vi "Differential Spikes chopper.vi"(4 "Spikes Array In":cluster{"Index":i32, "max value":sgl}[](array[cluster]), 5 "Analysis Info cluster In":T1={"Colour"=0, "Inst type"=enum."Pitot-static tube", "Inst name"="Manometer voltage", "Symbol"="U", "Code name"="", "Extra Info"="U", "Inst Array"=enum."PWA", "U"=0.0, "u^2"=0.0, "u^3"=0.0, "u^4"=0.0, "Skew_u"=0.0, "Kurt_u"=0.0, "Sd Error in Mean"=0.0, "% u'/U"=0.0, "X"=0.0, "Y"=0.0, "Z"=0.0, "Timescale integral Estimate"=0.0, "Sd Error in Variance"=0.0, "Calib File"=path "", "Calib Constants"=[], "Output Position"=FALSE, "Stats"=enum."None", "Av Sampling Rate"=0.0, "Av No of Samples"=0.0, "Total Meas Time (s)"=0.0, "OrigChName"="", "Max value"=0.0, "Min value"=0.0, "Req Sample Rate Hz"=0.0, "Sync Delay Time (s)"=0.0, "Ch No"=0, "Device"="", "Use Latest Calib"=FALSE, "Port"="", "Metadata Ch Names"=[], "Metadata Ch Values"=[], "Label"="", "chState"=enum."Solo", "Point Drift"=0.0, "inputConfig"=""} {"Kurt_u" format="%_3g"; "u^4" format="%_3g"; "u^3" format="%_3g"; "Sd Error in Variance" format="%_3g"; "u^2" format="%_3g"; "Sd Error in Mean" format="%_3g"; "U" format="%_3g"; "Sync Delay Time (s)" format="%.4f"; "Total Meas Time (s)" format="%_5g"; "Skew_u" format="%_3g"; "% u'/U" format="%_3g"}, 6 "Average Sampling Rate":sgl, 7 "C Trace":dbl[](array[numeric])) -> (0 "Spikes Array Out":cluster{"Index":i32, "max value":dbl}[](array[cluster]), 1 "No of Removed spikes":i32, 3 "Filtered Time Trace":sgl[](array[numeric]))   [LabVIEW 2022 SP3]
uses:
  Controls/Analysis_info_cluster.ctl
  Controls/Inst_type.ctl
  Controls/Instrument_Array.ctl
  Controls/channelState.ctl
panel:
  in  "Factor 2":sgl=2.5
  out "Min Spike Length":i32
  out "Spike Length":i32
  in  "Factor":sgl=1.5
  in  "p":sgl=0.97
  out "percentile":sgl
  out "Spike 2nd  All":sgl[](graph)
  out "Inst name":string
  in  "Play thro":bool
  out "Start time (Sec)":sgl
  in  "Display removed spikes":bool
  out "Potential spikes2":cluster{"Start Index":i32, "End Index":i32}[](array[cluster])
  out "Spikes1":cluster{"Start Index":i32, "End Index":i32}[](array[cluster])
  out "element":cluster{"Start Index":i32, "End Index":i32}
  in  "stop":bool
  in  "Desired index":i32 min=0
  out "Spike C":sgl[][](graph)
  out "Spike 2nd Derivative":sgl[](graph)
  out "Spikes 3":cluster{"Start Index":i32, "End Index":i32}[](array[cluster])
  out "C Threshold":sgl
  in  "Point info":cluster{"Start Index":i32, "End Index":i32}
  out "Derivative Theshold 1":sgl
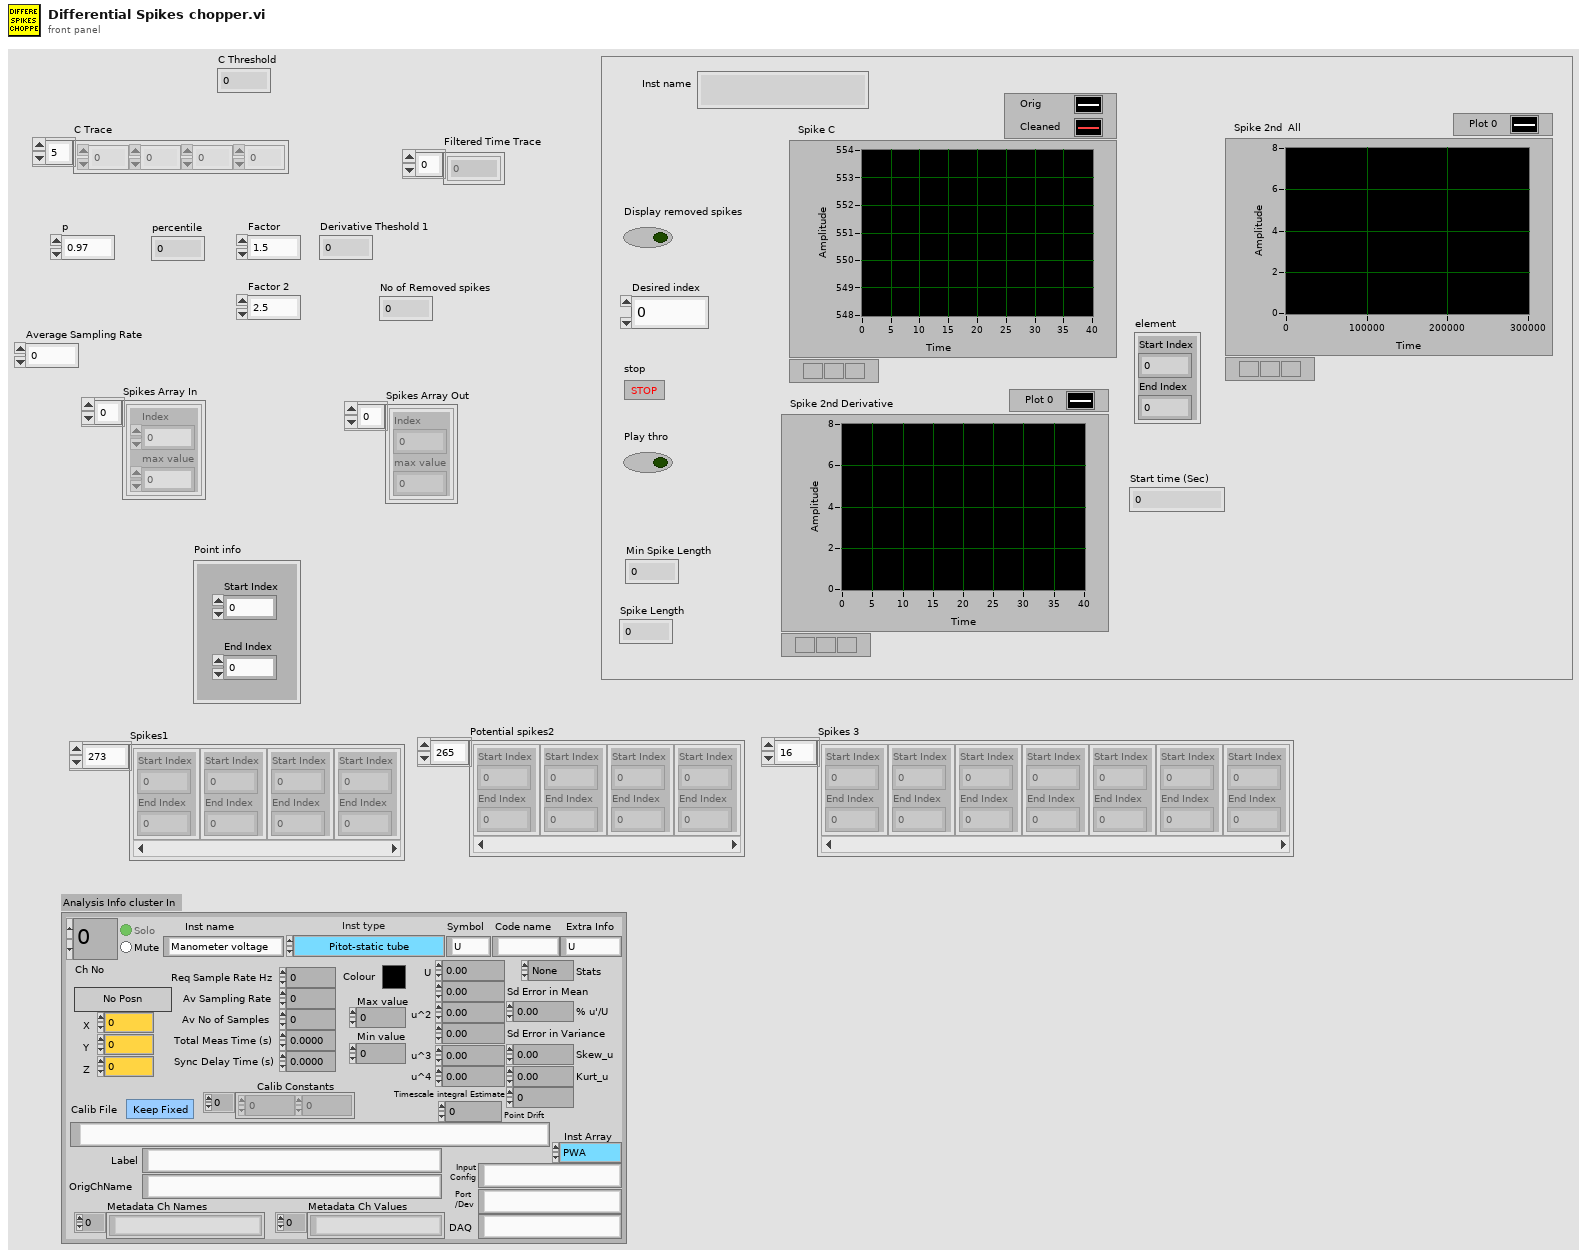
[diagram p1: front panel]
types:
  T1 = typedef "Analysis_info_cluster.ctl" = cluster{"Colour":u32, "Inst type":T2, "Inst name":string, "Symbol":string, "Code name":string, "Extra Info":string, "Inst Array":T3, "U":dbl, "u^2":dbl, "u^3":dbl, "u^4":dbl, "Skew_u":dbl, "Kurt_u":dbl, "Sd Error in Mean":dbl, "% u'/U":dbl, "X":dbl, "Y":dbl, "Z":dbl, "Timescale integral Estimate":dbl, "Sd Error in Variance":dbl, "Calib File":path, "Calib Constants":dbl[], "Output Position":bool, "Stats":enum16{"None", "Basic", "Full"}, "Av Sampling Rate":dbl, "Av No of Samples":dbl, "Total Meas Time (s)":dbl, "OrigChName":string, "Max value":dbl, "Min value":dbl, "Req Sample Rate Hz":dbl, "Sync Delay Time (s)":dbl, "Ch No":i16, "Device":string, "Use Latest Calib":bool, "Port":string, "Metadata Ch Names":string[], "Metadata Ch Values":string[], "Label":string, "chState":T4, "Point Drift":dbl, "inputConfig":string}
  T2 = typedef "Inst_type.ctl" = enum16{"Raw voltage", "Raw with zero offsetting", "Propeller anemometer", "Pressure Transducer", "Pitot-static tube", "Hot wire", "Cross wire 1", "Cross wire 2", "Generic Linear", "Generic Polynomial", "Generic BackPoly", "Fast FID", "Thermocouple", "Cold wire", "Pulsed Wire", "LDA Vel", "LDA Tran time", "LDA Arr time", "Microphone"}
  T3 = typedef "Instrument_Array.ctl" = enum16{"PWA", "LDA", "Analogue"}
  T4 = typedef "channelState.ctl" = enum32{"No Selection", "Solo", "Mute"}
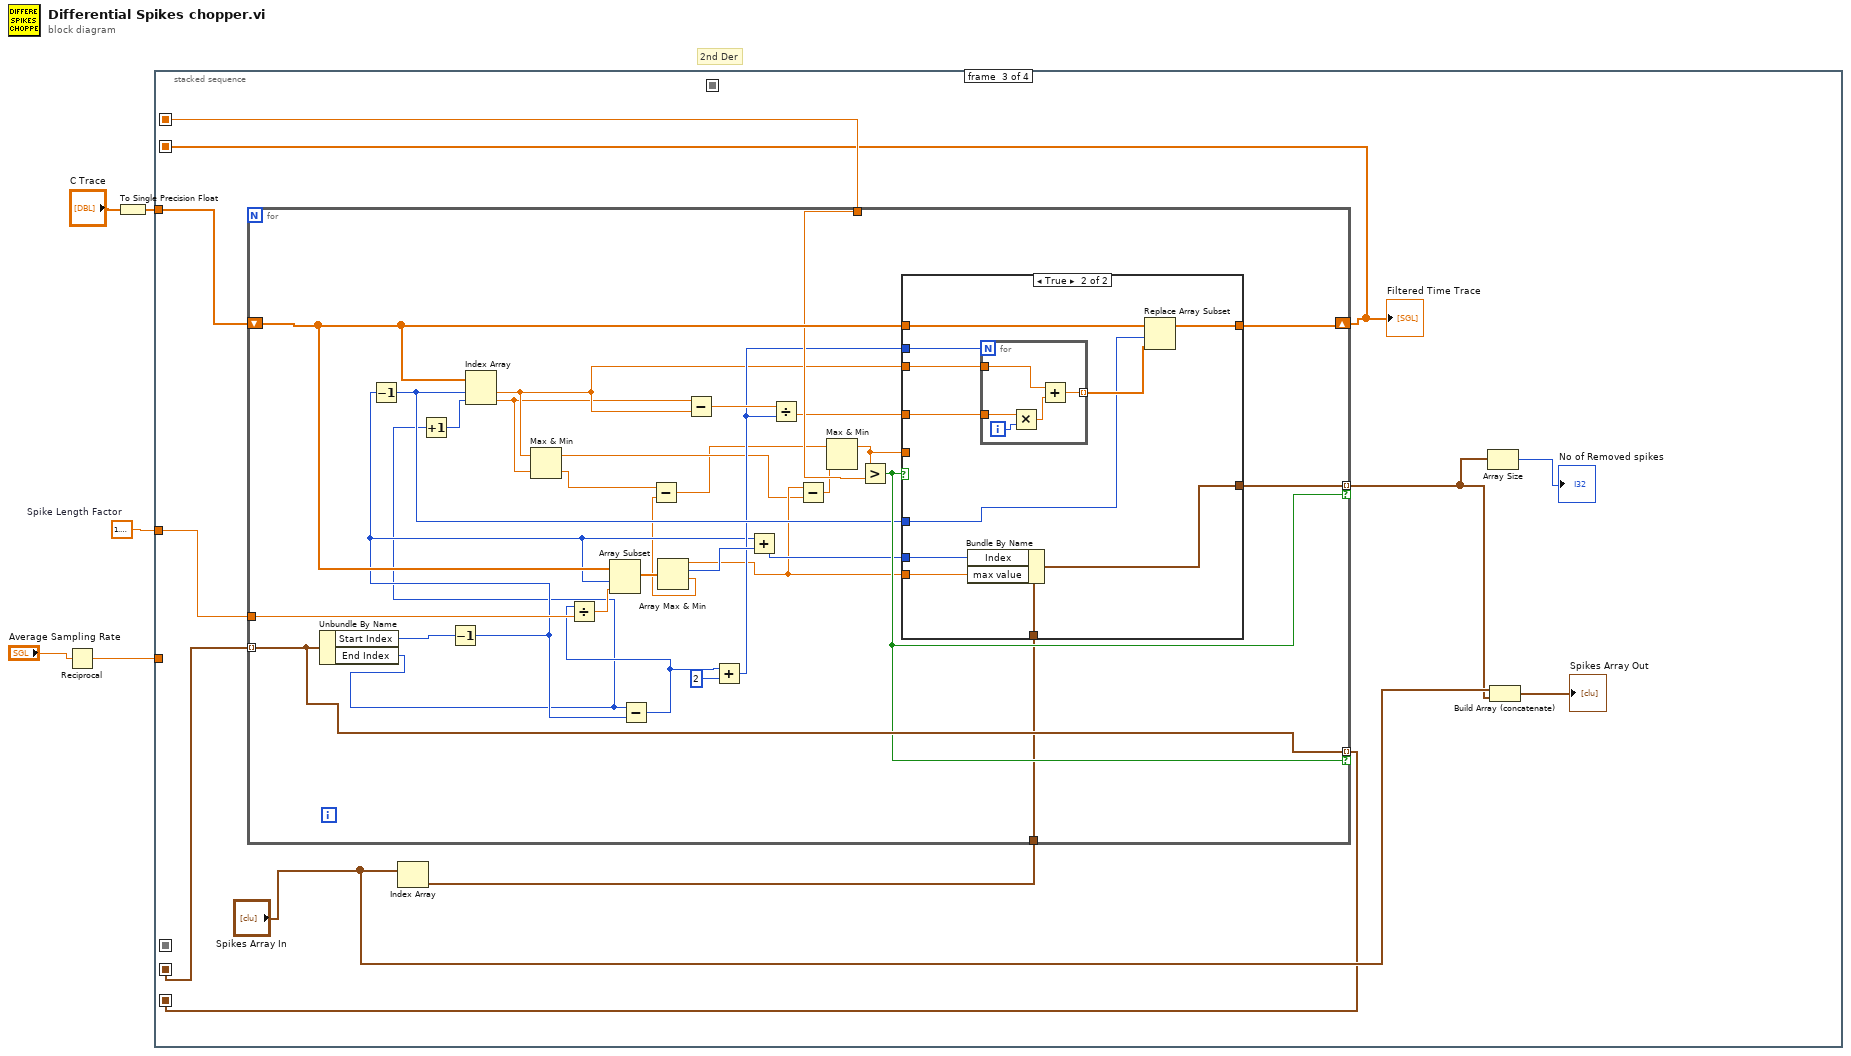
[diagram p0: block diagram]
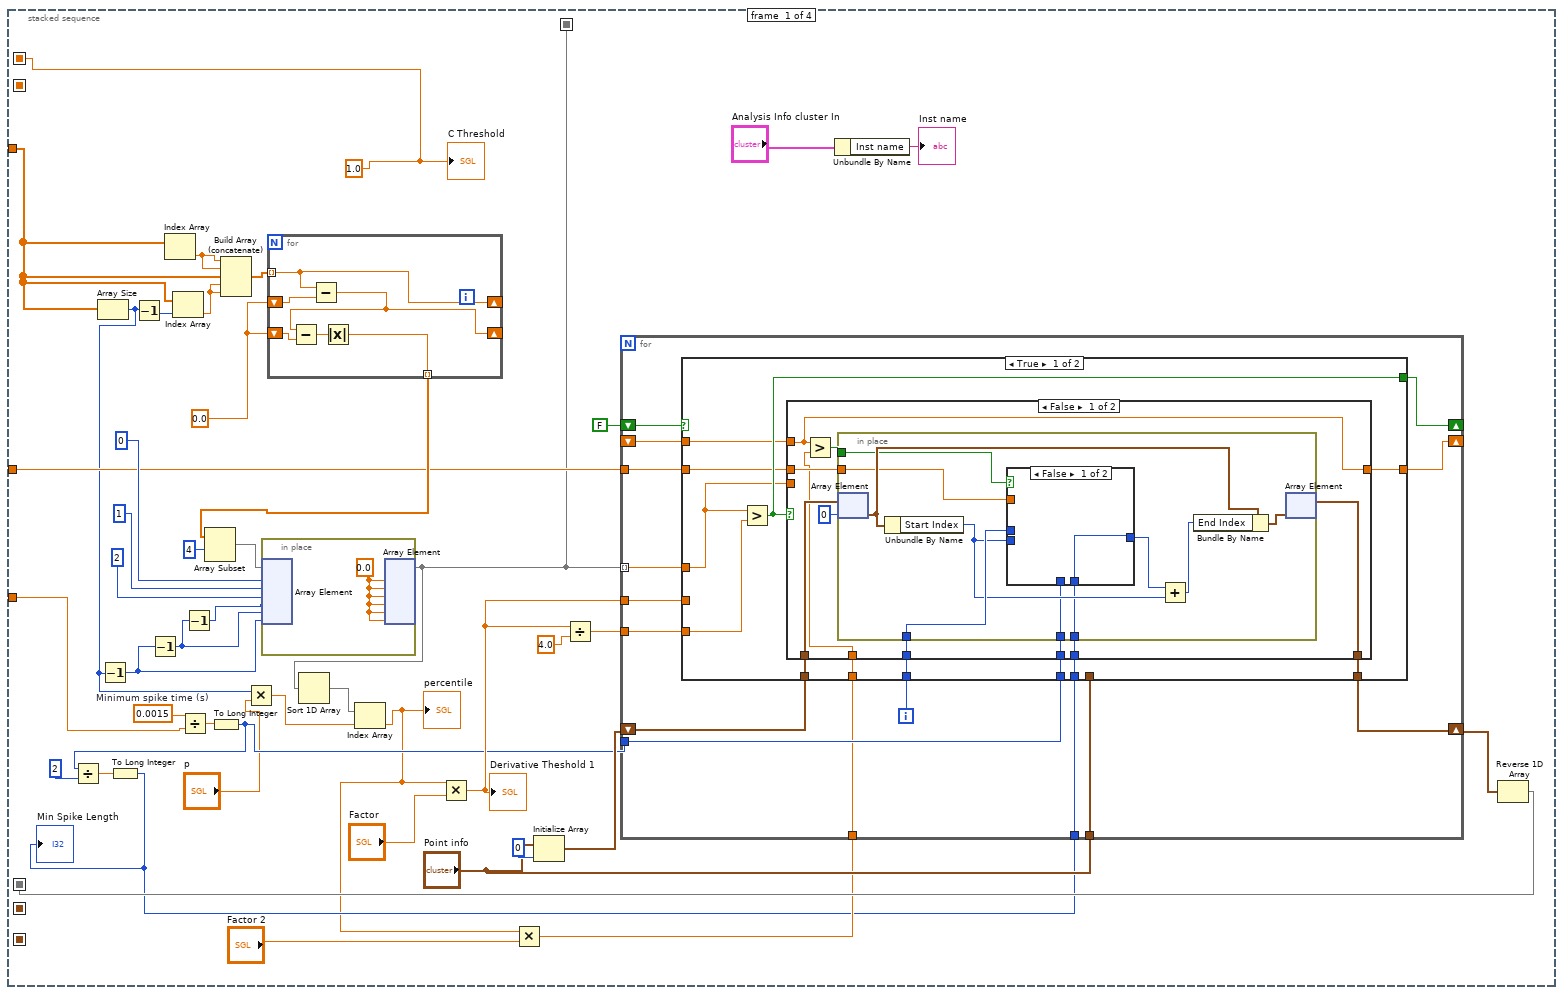
[diagram p2: hidden frame]
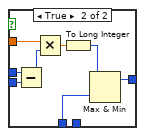
[diagram p3: hidden frame]
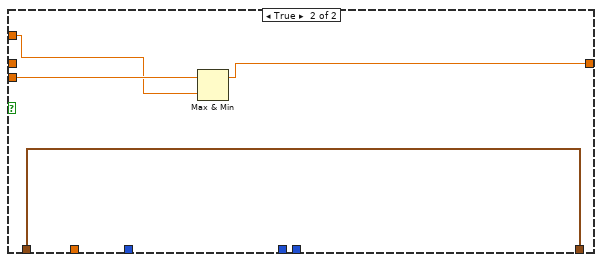
[diagram p4: hidden frame]
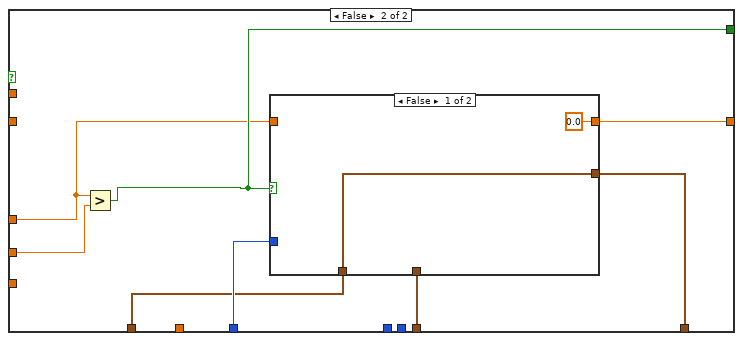
[diagram p5: hidden frame]
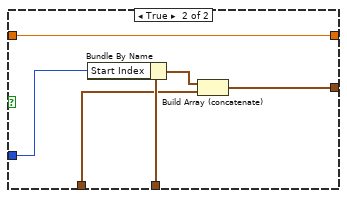
[diagram p6: hidden frame]
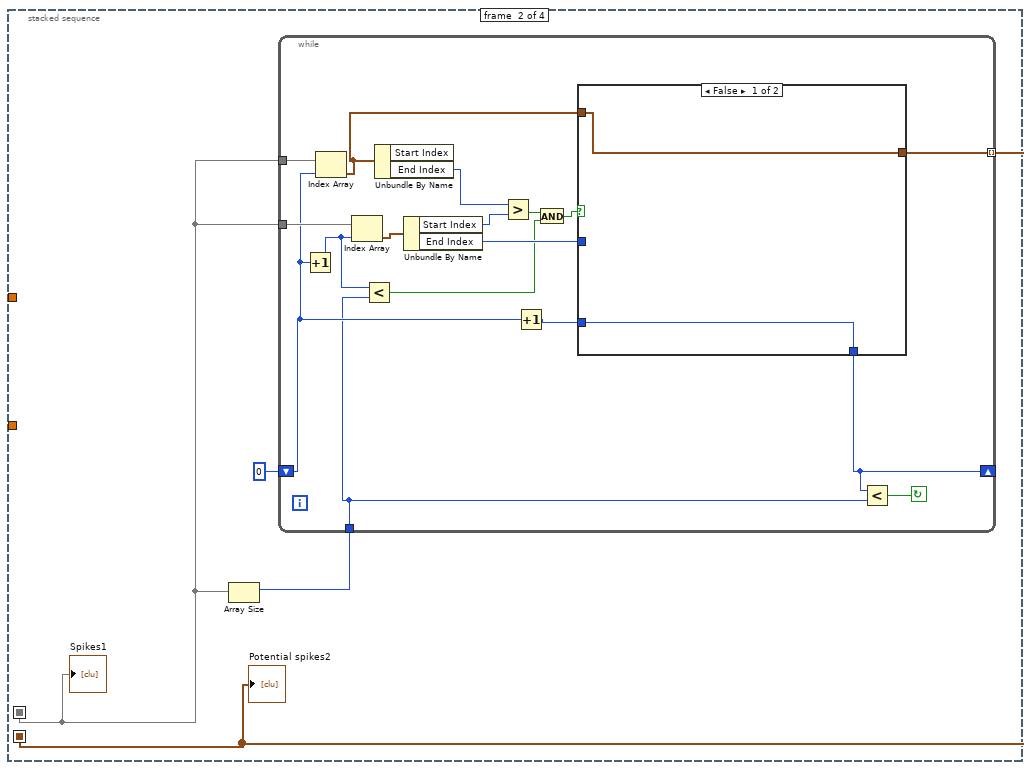
[diagram p7: hidden frame]
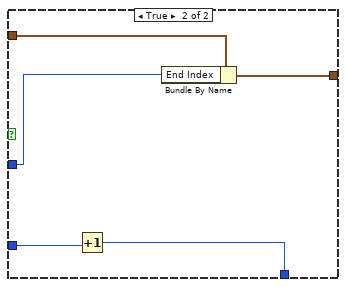
[diagram p8: hidden frame]
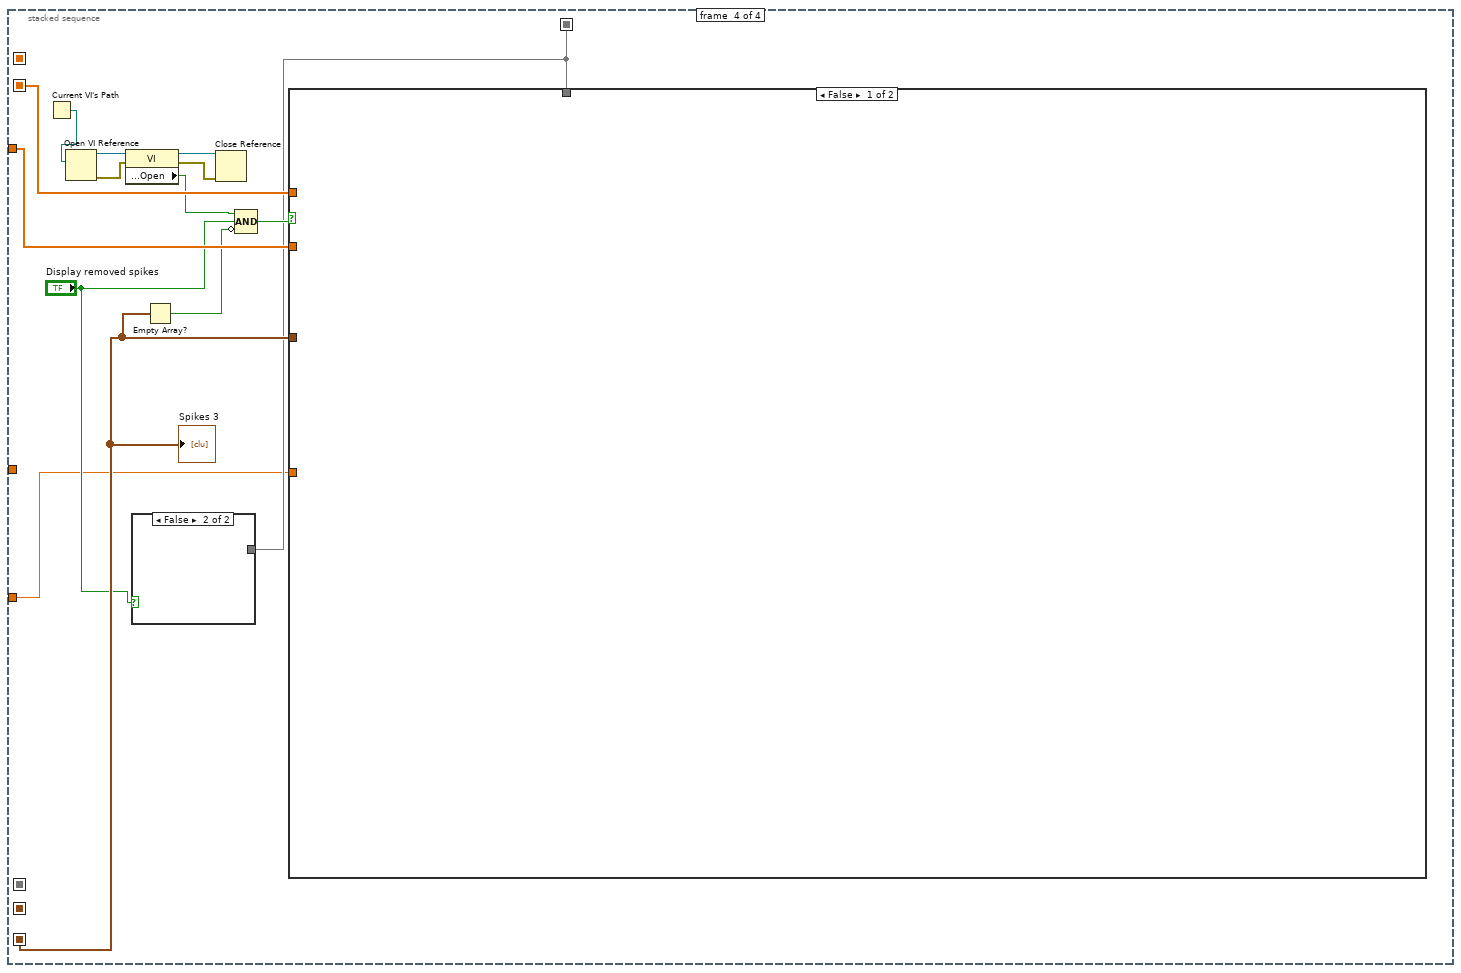
[diagram p10: hidden frame]
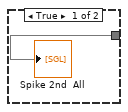
[diagram p11: hidden frame]
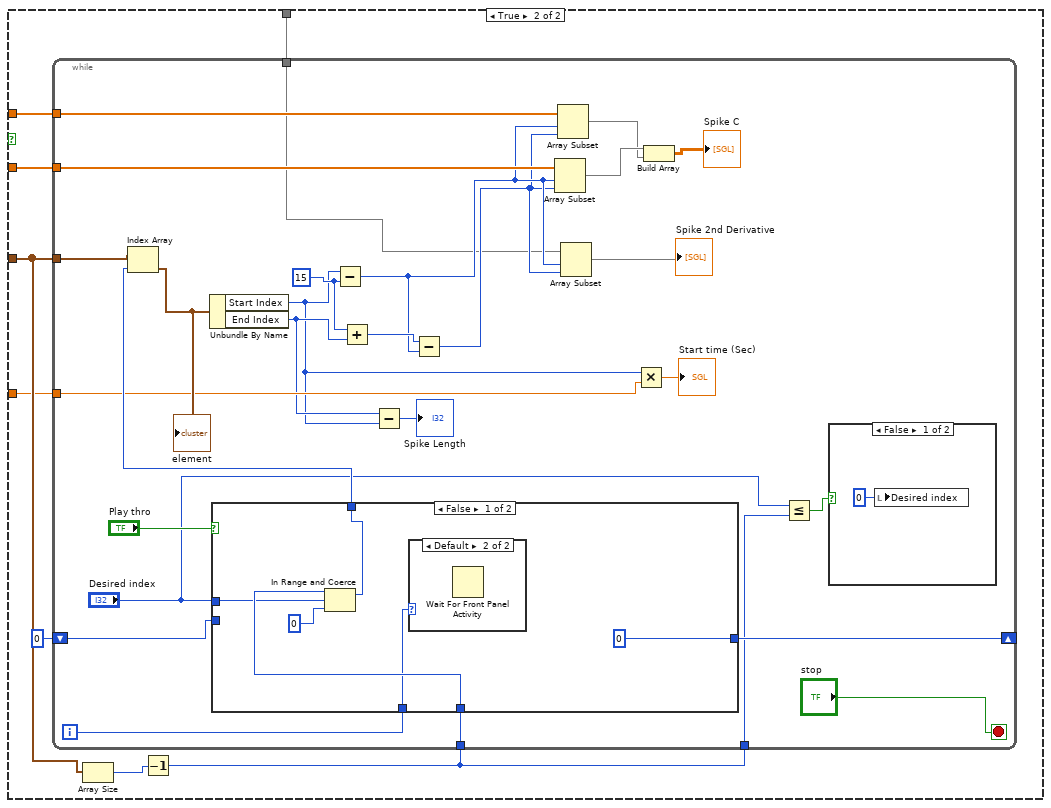
[diagram p12: hidden frame]
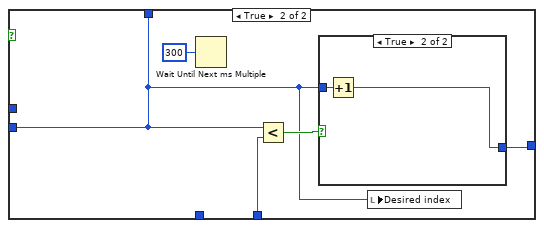
[diagram p15: hidden frame]
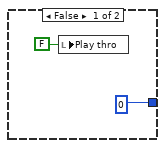
[diagram p16: hidden frame]
diagram:
  w4 = sgl 1.9  # Spike Length Factor
  # "2nd Der"
  n1 = Reciprocal(x="Average Sampling Rate") -> (1/x=w2:sgl)
  n2 = To Single Precision Float(number="C Trace") -> (single precision float=w1:sgl[])
  n3 = stacked-sequence {
    seq-local: [w29 _ _ _] -> [_ w135 _ _]
    seq-local: [w18 _ _ _] -> [_ _ w167 _]
    seq-local: [_ _ w164 _] -> [_ _ _ w226]
    seq-local: [_ _ w163 _] -> [_ _ _ w233]
    seq-local: [w11 _ _ _] -> [_ _ _ w222]
    seq-local: [_ w134 _ _] -> [_ _ w162 _]
    tunnel: w1 -> [w34 _ w171 w234]
    tunnel: w4 -> [w28 _ w161 _]
    tunnel: w2 -> [w20 _ _ w221]
    frame #0 {
      w18 = sgl 1.0 ("C Threshold")
      w21 = 0.0015  # Minimum spike time (s)
      w44 = sgl 0.0
      n4 = Array Size(array=w34) -> (size(s)=w9:i32)
      n5 = Decrement(x=w9) -> (x-1=w37:i32)
      n6 = Decrement(x=w9) -> (x-1=w46:i32)
      n7 = Decrement(x=w37) -> (x-1=w35:i32)
      n8 = Index Array(array=w34) -> (element=w47:sgl)  [unwired: 1 in]
      n9 = Index Array(array=w34, index=w46) -> (element=w45:sgl)
      n10 = Divide(x=w21, y=w20) -> (x/y=w19:dbl)
      n11 = Decrement(x=w35) -> (x-1=w36:i32)
      n12 = To Long Integer(number=w19) -> (32bit integer=w17:i32)
      n13 = Divide(x=w17, y=2) -> (x/y=w15:dbl)
      n14 = To Long Integer(number=w15) -> (32bit integer=w12:i32)
      "Min Spike Length" <- w12
      n15 = Build Array (concatenate)(w47, w47, w34, w45, w45) -> (w48:sgl[])
      n16 = Multiply(x=w9, y="p") -> (x*y=w7:sgl)
      n17 = for {
        shift-right: [w53] -> _
        shift-left: w44 -> [w56]
        tunnel: w48 -> [w53] mode=indexing
        tunnel: [w51] -> w39 mode=indexing
        shift-right: [w52] -> _
        shift-left: w44 -> [w55]
        n18 = Subtract(x=w53, y=w56) -> (x-y=w52:sgl)
        n19 = Subtract(x=w52, y=w55) -> (x-y=w54:sgl)
        n20 = Absolute Value(x=w54) -> (abs(x)=w51:sgl)
      }
      n21 = Array Subset(array=w39, index=4) -> (w38:sgl[])  [unwired: 1 in]
      n22 = in-place {
        w50 = sgl 0.0 ("element")
        n23 = in-place-array #1(w38, 0, 1, 2, w36, w35, w37) -> ()  [unwired: 6 out]
        n24 = in-place-array #1(w50, w50, w50, w50, w50, w50) -> (w11:sgl[])  [unwired: 6 out]
      }
      n25 = Sort 1D Array(array=w11) -> (sorted array=w8:sgl[])
      n26 = Index Array(array=w8, index=w7) -> (element=w6:sgl)
      "percentile" <- w6
      n27 = Multiply(x=w6, y="Factor") -> (x*y=w24:sgl)
      "Derivative Theshold 1" <- w24
      n28 = Multiply(x=w6, y="Factor 2") -> (x*y=w13:sgl)
      n29 = Initialize Array("Point info", 0 ("dimension size")) -> (w32:cluster{"Start Index":i32, "End Index":i32}[])
      n30 = Divide(x=w24, y=sgl 4.0) -> (x/y=w23:sgl)
      n31 = for {
        shift-right: [w67] -> _
        shift-left: FALSE -> [w70]
        tunnel: w11 -> [w71] mode=indexing
        tunnel: w24 -> [w69]
        shift-right: [w64] -> w30
        shift-left: w32 -> [w65]
        tunnel: "Point info" -> [w66]
        tunnel: w28 -> [w63]
        tunnel: w23 -> [w62]
        tunnel: w17 -> [w61]
        shift-right: [w60] -> _
        shift-left: _ -> [w59]
        tunnel: w13 -> [w58]
        tunnel: w12 -> [w57]
        i -> [w68]
        n32 = case shown="True" w70 {
          tunnel: [w80 w119] -> w67
          tunnel: w71 -> [w76 w117]
          tunnel: w69 -> [_ w124]
          tunnel: w68 -> [w81 w123]
          tunnel: w66 -> [_ w122]
          tunnel: w65 -> [w83 w121]
          tunnel: [w82 w120] -> w64
          tunnel: w63 -> [w79 _]
          tunnel: w62 -> [w78 _]
          tunnel: w61 -> [w77 _]
          tunnel: [w74 w118] -> w60
          tunnel: w59 -> [w75 _]
          tunnel: w58 -> [w73 _]
          tunnel: w57 -> [w72 _]
          frame True {
            n33 = Greater?(x=w76, y=w78) -> (0:w80:bool)
            n34 = case shown="False" w80 {
              tunnel: w81 -> [w89 _]
              tunnel: w83 -> [w93 w116]
              tunnel: [w92 w116] -> w82
              tunnel: w79 -> [w90 _]
              tunnel: w77 -> [w88 _]
              tunnel: w76 -> [_ w115]
              tunnel: w75 -> [w84 w114]
              tunnel: [w84 w113] -> w74
              tunnel: w73 -> [w87 _]
              tunnel: w72 -> [w85 _]
              frame False {
                n35 = Greater?(x=w84, y=w87) -> (0:w86:bool)
                n36 = in-place {
                  in-place-border: w90 -> [w101]
                  in-place-border: w89 -> [w100]
                  in-place-border: w88 -> [w97]
                  in-place-border: w86 -> [w95]
                  in-place-border: w85 -> [w94]
                  n37 = in-place-array #2(w93, 0) -> (w103:cluster{"Start Index":i32, "End Index":i32})
                  n38 = Unbundle By Name(w103) -> ("Start Index"=w99:i32)
                  n39 = case shown="False" w95 {
                    tunnel: w101 -> [_ w110]
                    tunnel: w100 -> [_ w109]
                    tunnel: w99 -> [_ w108]
                    tunnel: w97 -> [_ w106]
                    tunnel: [w104 w105] -> w96
                    tunnel: w94 -> [w104 _]
                    frame False {
                    }
                    frame True {
                      n40 = Subtract(x=w109, y=w108) -> (x-y=w111:i32)
                      n41 = Multiply(x=w110, y=w111) -> (x*y=w112:sgl)
                      n42 = To Long Integer(number=w112) -> (32bit integer=w107:i32)
                      n43 = Max & Min(x=w107, y=w106) -> (max(x,y)=w105:i32)  [unwired: 1 out]
                    }
                  }
                  n44 = Add(x=w96, y=w99) -> (x+y=w98:i32)
                  n45 = Bundle By Name(cluster=w103, "End Index"=w98) -> (w102:cluster{"Start Index":i32, "End Index":i32})
                  n46 = in-place-array #2(w102) -> (w92:cluster{"Start Index":i32, "End Index":i32}[])  [unwired: 1 out]
                }
              }
              frame True {
                n47 = Max & Min(x=w115, y=w114) -> (max(x,y)=w113:sgl)  [unwired: 1 out]
              }
            }
          }
          frame False {
            n48 = Greater?(x=w117, y=w124) -> (0:w119:bool)
            n49 = case shown="False" w119 {
              tunnel: w123 -> [_ w132]
              tunnel: w122 -> [_ w130]
              tunnel: w121 -> [w126 w129]
              tunnel: [w126 w128] -> w120
              tunnel: [sgl 0.0 w127] -> w118
              tunnel: w117 -> [_ w127]
              frame False {
              }
              frame True {
                n50 = Bundle By Name(cluster=w130, "Start Index"=w132) -> (w131:cluster{"Start Index":i32, "End Index":i32})
                n51 = Build Array (concatenate)(w131, w129) -> (w128:cluster{"Start Index":i32, "End Index":i32}[])
              }
            }
          }
        }
      }
      n52 = Unbundle By Name("Analysis Info cluster In") -> ("Inst name"=→"Inst name":string)
      n53 = Reverse 1D Array(array=w30) -> (reversed array=w29:cluster{"Start Index":i32, "End Index":i32}[])
      "C Threshold" <- w18
    }
    frame #1 {
      n54 = Array Size(array=w135) -> (size(s)=w133:i32)
      n55 = while {
        tunnel: w135 -> [w146]
        tunnel: w135 -> [w153]
        tunnel: [w148] -> w134 mode=indexing
        shift-right: [w143] -> _
        shift-left: 0 -> [w145]
        tunnel: w133 -> [w137]
        stop <- w142 continue-if-true
        n56 = Increment(x=w145) -> (x+1=w141:i32)
        n57 = Index Array(array=w146, index=w145) -> (element=w147:cluster{"Start Index":i32, "End Index":i32})
        n58 = Index Array(array=w153, index=w141) -> (element=w152:cluster{"Start Index":i32, "End Index":i32})
        n59 = Less?(x=w141, y=w137) -> (x < y?=w139:bool)
        n60 = Unbundle By Name(w147) -> ("End Index"=w151:i32)  [unwired: 1 out]
        n61 = Unbundle By Name(w152) -> ("Start Index"=w150:i32, "End Index"=w149:i32)
        n62 = Greater?(x=w151, y=w150) -> (0:w140:bool)
        n63 = Increment(x=w145) -> (x+1=w144:i32)
        n64 = And(x=w140, y=w139) -> (x .and. y?=w138:bool)
        n65 = case shown="False" w138 {
          tunnel: w147 -> [w154 w160]
          tunnel: w149 -> [_ w159]
          tunnel: [w154 w158] -> w148
          tunnel: [w155 w156] -> w143
          tunnel: w144 -> [w155 w157]
          frame False {
          }
          frame True {
            n66 = Increment(x=w157) -> (x+1=w156:i32)
            n67 = Bundle By Name(cluster=w160, "End Index"=w159) -> (w158:cluster{"Start Index":i32, "End Index":i32})
          }
        }
        n68 = Less?(x=w143, y=w137) -> (x < y?=w142:bool)
      }
      "Potential spikes2" <- w134
      "Spikes1" <- w135
    }
    frame #2 {
      n69 = Index Array(array="Spikes Array In") -> (element=w170:cluster{"Index":i32, "max value":sgl})  [unwired: 1 in]
      n70 = for {
        shift-right: [w200] -> w163
        shift-left: w171 -> [w201]
        tunnel: w162 -> [w199] mode=indexing
        tunnel: w170 -> [w195]
        tunnel: [w202] -> w166 mode=indexing if=w196
        tunnel: w167 -> [w197]
        tunnel: [w199] -> w164 mode=indexing if=w196
        tunnel: w161 -> [w198]
        n71 = Unbundle By Name(w199) -> ("Start Index"=w172:i32, "End Index"=w173:i32)
        n72 = Increment(x=w173) -> (x+1=w194:i32)
        n73 = Decrement(x=w172) -> (x-1=w181:i32)
        n74 = Decrement(x=w181) -> (x-1=w188:i32)
        n75 = Index Array(array=w201, index #1=w188, index #2=w194) -> (element #1=w185:sgl, element #2=w184:sgl)
        n76 = Max & Min(x=w185, y=w184) -> (max(x,y)=w182:sgl, min(x,y)=w178:sgl)
        n77 = Subtract(x=w173, y=w181) -> (x-y=w180:i32)
        n78 = Divide(x=w180, y=w198) -> (x/y=w179:sgl)
        n79 = Array Subset(array=w201, index=w181, length=w179) -> (w191:sgl[])
        n80 = Array Max & Min(array=w191) -> (max value=w183:sgl, max index (indices)=w190:i32, min value=w177:sgl)  [unwired: 1 out]
        n81 = Subtract(x=w178, y=w177) -> (x-y=w176:sgl)
        n82 = Subtract(x=w184, y=w185) -> (x-y=w193:sgl)
        n83 = Add(x=w180, y=2) -> (x+y=w186:i32)
        n84 = Add(x=w181, y=w190) -> (x+y=w189:i32)
        n85 = Divide(x=w193, y=w186) -> (x/y=w192:sgl)
        n86 = Subtract(x=w183, y=w182) -> (x-y=w175:sgl)
        n87 = Max & Min(x=w176, y=w175) -> (max(x,y)=w174:sgl)  [unwired: 1 out]
        n88 = Greater?(x=w174, y=w197) -> (0:w196:bool)
        n89 = case shown="True" w196 {
          tunnel: w195 -> [w203 w215]
          tunnel: [w203 w214] -> w202
          tunnel: w192 -> [_ w213]
          tunnel: w201 -> [w204 w212]
          tunnel: [w204 w210] -> w200
          tunnel: w189 -> [_ w209]
          tunnel: w188 -> [_ w208]
          tunnel: w186 -> [_ w207]
          tunnel: w185 -> [_ w206]
          tunnel: w183 -> [_ w205]
          tunnel: w174 -> [_ _]
          frame False {
          }
          frame True {
            n90 = Bundle By Name(cluster=w215, "Index"=w209, "max value"=w205) -> (w214:cluster{"Index":i32, "max value":sgl})
            n91 = for {
              N: w207 -> [_]
              tunnel: w213 -> [w219]
              tunnel: w206 -> [w217]
              tunnel: [w216] -> w211 mode=indexing
              i -> [w220]
              n92 = Multiply(x=w219, y=w220) -> (x*y=w218:sgl)
              n93 = Add(x=w217, y=w218) -> (x+y=w216:sgl)
            }
            n94 = Replace Array Subset(array=w212, new element=w211, index=w208) -> (w210:sgl[])
          }
        }
      }
      "Filtered Time Trace" <- w163
      n95 = Array Size(array=w166) -> (size(s)=→"No of Removed spikes":i32)
      n96 = Build Array (concatenate)("Spikes Array In", w166) -> (→"Spikes Array Out":cluster{"Index":i32, "max value":sgl}[])
    }
    frame #3 {
      n97 = Current VI's Path() -> (path=w230:path)
      n98 = Open VI Reference(vi path=w230) -> (vi reference=w232:refnum<vi>, error out=w231:errorcluster)  [unwired: 1 in, 4 out]
      n99 = property class="VI"(reference=w232, error in=w231) -> (reference out=w229:refnum<vi>, error out=w228:errorcluster, "Front Panel Window:Open"=w225:bool)
      n100 = case shown="False" "Display removed spikes" {
        tunnel: w222 -> [w235 _]
        frame True {
          "Spike 2nd  All" <- w235
        }
        frame False {
        }
      }
      n101 = Empty Array?(array=w226) -> (empty?=w224:bool)
      n102 = Close Reference(reference=w229, error in (no error)=w228) -> ()  [unwired: 1 out]
      n103 = Compound Arithmetic op=AND(w225, "Display removed spikes", invert w224) -> (w227:bool)
      n104 = case shown="False" w227 {
        tunnel: w234 -> [_ w243]
        tunnel: w233 -> [_ w242]
        tunnel: w222 -> [_ w241]
        tunnel: w226 -> [_ w240]
        tunnel: w221 -> [_ w236]
        frame False {
        }
        frame True {
          n105 = Array Size(array=w240) -> (size(s)=w239:i32)
          n106 = Decrement(x=w239) -> (x-1=w237:i32)
          n107 = while {
            tunnel: w240 -> [w271]
            tunnel: w243 -> [w267]
            tunnel: w242 -> [w266]
            tunnel: w241 -> [w248]
            shift-right: [w257] -> _
            shift-left: 0 ("f") -> [w258]
            tunnel: w237 -> [w259]
            tunnel: w237 -> [w254]
            tunnel: w236 -> [w247]
            i -> [w249]
            stop <- "stop" stop-if-true
            w269 = 15 ("y")
            n108 = case shown="False" "Play thro" {
              tunnel: w258 -> [_ w279]
              tunnel: [w275 w279] -> w260
              tunnel: w259 -> [w277 w283]
              tunnel: [0 ("f") w280] -> w257
              tunnel: "Desired index" -> [w274 _]
              tunnel: w249 -> [w273 _]
              frame False {
                n109 = In Range and Coerce(upper limit=w277, x=w274, lower limit=0) -> (coerced(x)=w275:i32)  [unwired: 1 out]
                n110 = case shown="Default" w273 {
                  frame 0 {
                  }
                  frame Default {
                    n111 = Wait For Front Panel Activity() -> ()  [unwired: 3 in, 1 out]
                  }
                }
              }
              frame True {
                n112 = Wait Until Next ms Multiple(millisecond multiple=u32 300) -> ()  [unwired: 1 out]
                n113 = Less?(x=w279, y=w283) -> (x < y?=w281:bool)
                n114 = case shown="True" w281 {
                  tunnel: w279 -> [_ w287]
                  tunnel: [0 ("f") w286] -> w280
                  frame False {
                    n115 = local write "Play thro"(FALSE ("Play thro")) -> ()
                  }
                  frame True {
                    n116 = Increment(x=w287) -> (x+1=w286:i32)
                  }
                }
                n117 = local write "Desired index"(w279) -> ()
              }
            }
            n118 = Index Array(array=w271, index=w260) -> (element=w270:cluster{"Start Index":i32, "End Index":i32})
            "element" <- w270
            n119 = Unbundle By Name(w270) -> ("Start Index"=w245:i32, "End Index"=w246:i32)
            n120 = Subtract(x=w245, y=w269) -> (x-y=w251:i32)
            n121 = Add(x=w269, y=w246) -> (x+y=w268:i32)
            n122 = Subtract(x=w246, y=w245) -> (x-y=→"Spike Length":i32)
            n123 = Subtract(x=w268, y=w251) -> (x-y=w250:i32)
            n124 = Array Subset(array=w267, index=w251, length=w250) -> (w263:sgl[])
            n125 = Array Subset(array=w266, index=w251, length=w250) -> (w262:sgl[])
            n126 = Array Subset(array=w248, index=w251, length=w250) -> (→"Spike 2nd Derivative":sgl[])
            n127 = Multiply(x=w245, y=w247) -> (x*y=→"Start time (Sec)":sgl)
            n128 = Build Array(w263, w262) -> (→"Spike C":sgl[][])
            n129 = Less Or Equal?(x="Desired index", y=w254) -> (x <= y?=w253:bool)
            n130 = case shown="False" w253 {
              frame False {
                n131 = local write "Desired index"(0 ("Desired index")) -> ()
              }
              frame True {
              }
            }
          }
        }
      }
      "Spikes 3" <- w226
    }
  }
